vi "InitializeNetworkStreamWriter.vi"(11 "Boat Type":T1) -> (0 "error out":errorcluster, 3 "NetworkStreamWriter out":refnum<class "NetworkStreamWriter.lvclass">)   [LabVIEW 2013]
doc: "Initializes the Writer network stream."
uses:
  RIO-OCU_Comm/NetworkStreams/Writer/NetworkStreamWriter.lvclass
  cRIO_Code/Data/TypeDefs/BoatType.ctl
  RIO-OCU_Comm/ToRIO.ctl
  CommandMessages.ctl
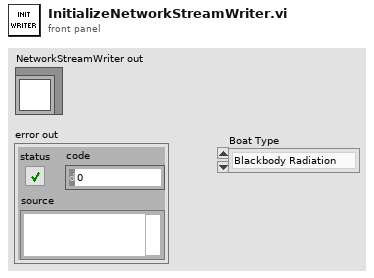
[diagram p1: front panel]
types:
  T1 = typedef "BoatType.ctl" = enum16{"Blackbody Radiation", "ReadLog", "Little boats", "Simulation", "Damn Yankee"}
  T2 = typedef "CommandMessages.ctl" = enum16{"Pass", "OverrideMode", "Add mission", "Delete mission", "Add obstacle", "Delete obstacle", "Change constants", "Check mission ID", "Check obstacle ID"}
  T3 = typedef "ToRIO.ctl" = cluster{"Commands":T2, "Variant":variant}
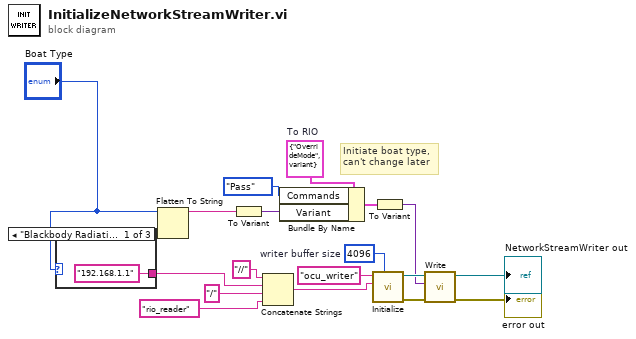
[diagram p0: block diagram]
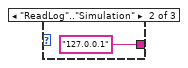
[diagram p2: hidden frame]
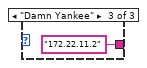
[diagram p3: hidden frame]
diagram:
  w8 = T3 {"Commands"=enum."OverrideMode", "Variant"=variant}  # To RIO
  w3 = 4096  # writer buffer size
  # "Initiate boat type,\ncan't change later"
  n1 = case shown="\"Blackbody Radiation\", Default" "Boat Type" {
    tunnel: ["192.168.1.1" "127.0.0.1" "172.22.11.2"] -> w1
    frame "Blackbody Radiation", Default {
    }
    frame "ReadLog".."Simulation" {
    }
    frame "Damn Yankee" {
    }
  }
  n2 = Flatten To String(anything="Boat Type") -> (data string=w18:string)  [unwired: 3 in, 2 out]
  n3 = To Variant(anything=w18) -> (Variant=w16:variant)
  n4 = Concatenate Strings("//" ("string"), w1, "/", "rio_reader" ("string")) -> (w5:string)
  n5 = Bundle By Name(cluster=w8, "Commands"=CommandMessages."Pass", "Variant"=w16) -> (w17:T3)
  n6 = call "Initialize.vi"("writer buffer size"=w3, "reader url"=w5, "writer name"="ocu_writer") -> ("error out"=w12:errorcluster, "NetworkStreamWriter out"=w11:refnum<class "NetworkStreamWriter.lvclass">)  [unwired: 7 in]
  n7 = To Variant(anything=w17) -> (Variant=w9:variant)
  n8 = call "Write.vi"("error in (no error)"=w12, "element"=w9, "NetworkStreamWriter in"=w11) -> ("error out"=→"error out":errorcluster, "NetworkStreamWriter out"=→"NetworkStreamWriter out":refnum<class "NetworkStreamWriter.lvclass">)  [unwired: 7 in]
